vi "Write Time.vi"(8 "error in (no error)":errorcluster, 10 "Time Stamp":timestamp, 11 "Shutter in":refnum<class "Shutter.lvclass">) -> (0 "error out":errorcluster, 3 "Shutter out":refnum<class "Shutter.lvclass">)   [LabVIEW 2016, in "Shutter.lvclass"]
uses:
  Shutter.lvclass
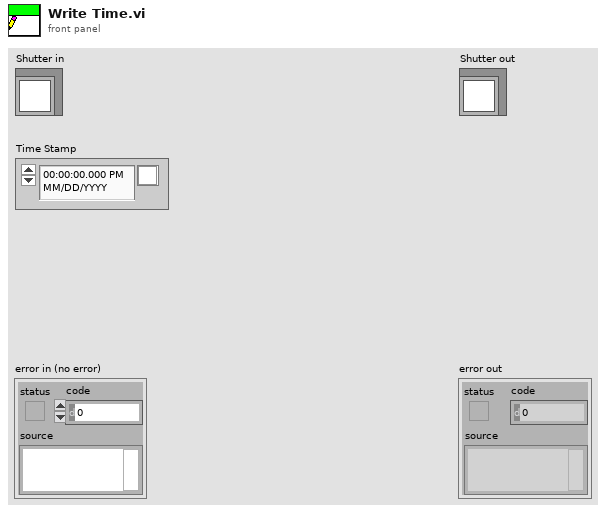
[diagram p1: front panel]
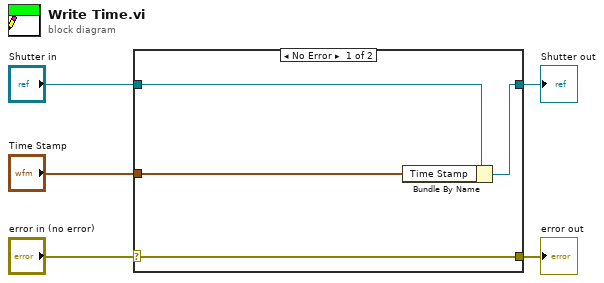
[diagram p0: block diagram]
diagram:
  n1 = case shown="No Error" "error in (no error)" {
    selector: "error in (no error)" -> [w9 w10]
    tunnel: [w9 w10] -> w4
    tunnel: [w7 w11] -> w2
    tunnel: "Shutter in" -> [w8 w11]
    tunnel: "Time Stamp" -> [w6 _]
    frame No Error {
      n2 = Bundle By Name(cluster=w8, "Time Stamp"=w6) -> (w7:refnum<class "Shutter.lvclass">)
    }
    frame Error {
    }
  }
  "error out" <- w4
  "Shutter out" <- w2
